vi "I2C config.vi"(4 "Clock Rate":u32=1000, 6 "FPGA Clock (40 MHz)":u32=40000000, 7 "Port Number":u8, 8 "error in (no error)":errorcluster, 9 "Address Type (7-bit)":enum16{"7-bit", "10-bit"}(ring), 10 "Address":u16=25, 11 "FPGA VI Reference":refnum<k20>) -> (0 "error out":errorcluster, 3 "FPGA Information Out":T1)   [LabVIEW 2012]
uses:
  <vilib>/IEDriver/SPIandI2C/Host/I2C/I2C Host.lvlib
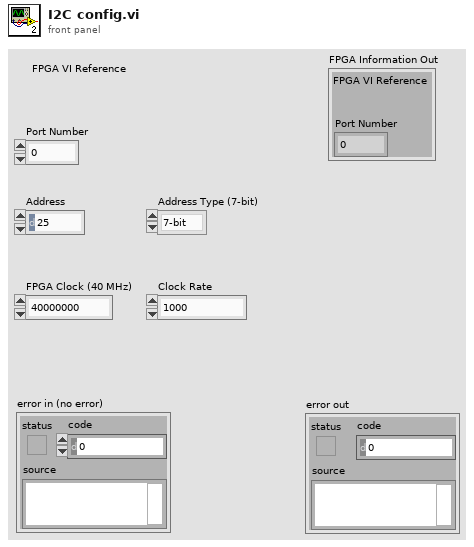
[diagram p1: front panel]
types:
  T1 = cluster{"FPGA VI Reference":refnum<k20>, "Port Number":u8}
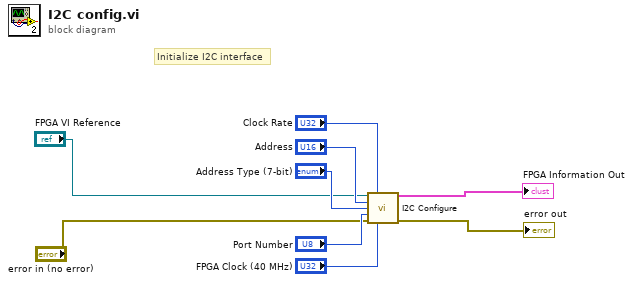
[diagram p0: block diagram]
diagram:
  # "Initialize I2C interface"
  n1 = call <vilib>:"I2C Configure.vi"("FPGA VI Reference"="FPGA VI Reference", "Clock Rate"="Clock Rate", "Address"="Address", "Address Type (7-bit)"="Address Type (7-bit)", "Port Number"="Port Number", "error in (no error)"="error in (no error)", "FPGA Clock (40 MHz)"="FPGA Clock (40 MHz)") -> ("FPGA Information Out"=→"FPGA Information Out":T1, "error out"=→"error out":errorcluster)  [unwired: 7 in]
